vi "Type Conversion.From Double (I16).vi"(3 "value in":dbl) -> (1 "value out":i16)   [LabVIEW 2016, in "VeriStand Data.lvlib"]
doc: "Converts the provided double float values to the specified data type, preserving the numerical value of the data."
uses:
  VeriStand Data.lvlib
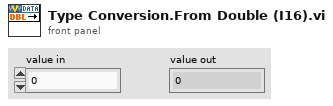
[diagram p1: front panel]
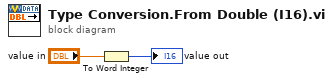
[diagram p0: block diagram]
diagram:
  n1 = To Word Integer(number="value in") -> (16bit integer=→"value out":i16)
